vi "Emulator.vi"() -> ()   [LabVIEW 2014]
uses:
  <vilib>/Utility/file.llb/Read From Spreadsheet File (string).vi
panel:
  out "Error Out":errorcluster
  in  "Error In":errorcluster
  in  "Write Loop stop":bool
  in  "file path (dialog if empty)":path=path "C:/Ehsan Temp Folder/TFS/LV/Data Logging with LabVIEW/SV names.csv"
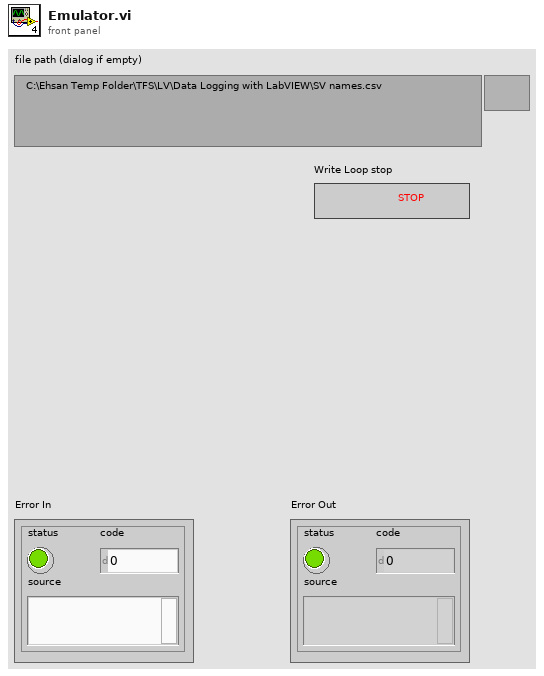
[diagram p1: front panel]
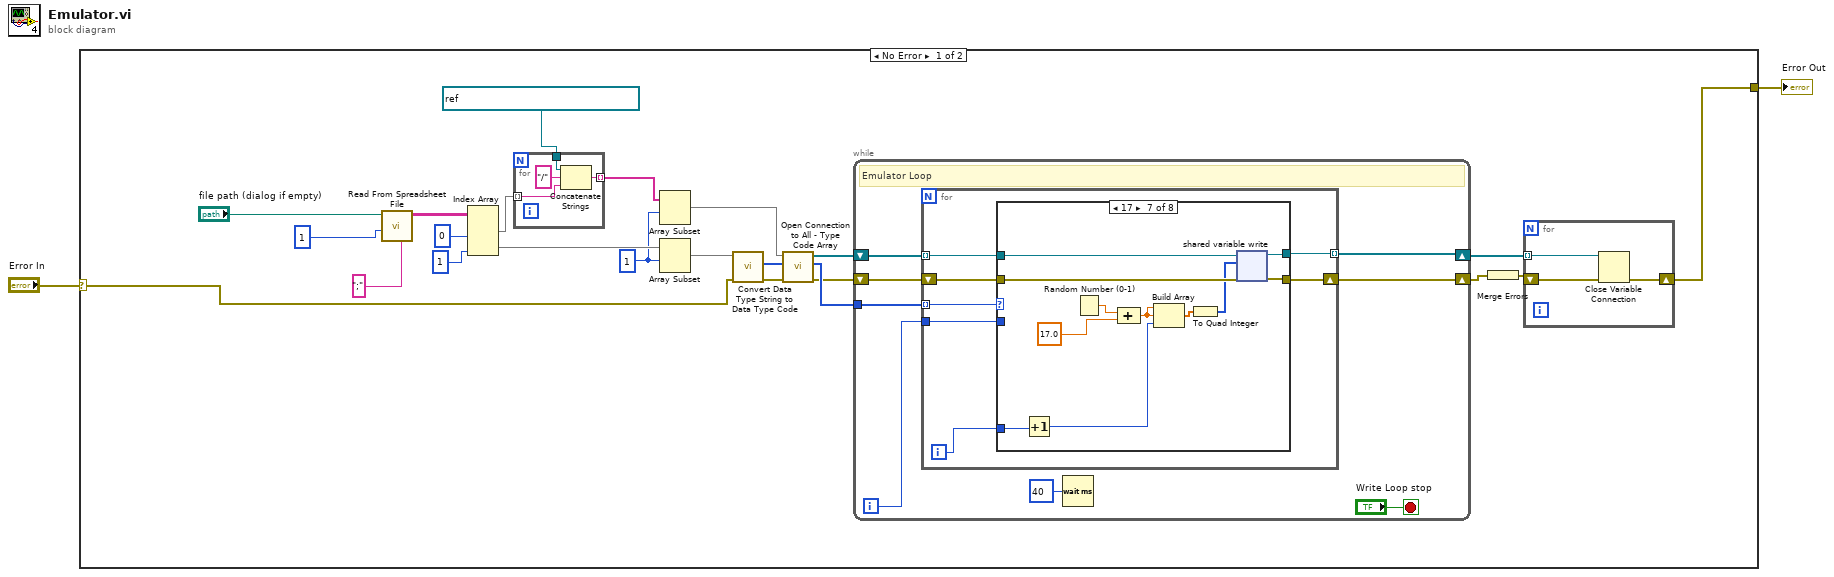
[diagram p0: block diagram]
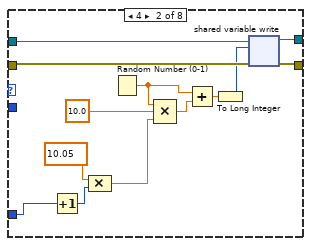
[diagram p3: hidden frame]
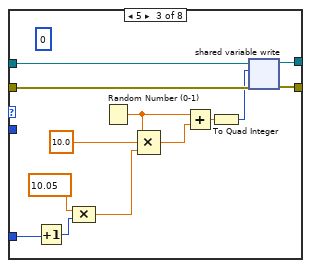
[diagram p4: hidden frame]
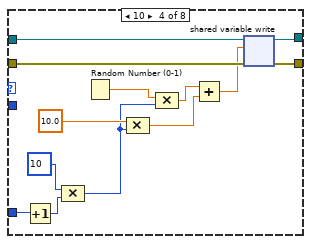
[diagram p5: hidden frame]
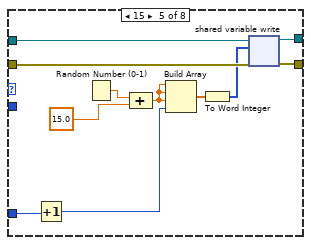
[diagram p6: hidden frame]
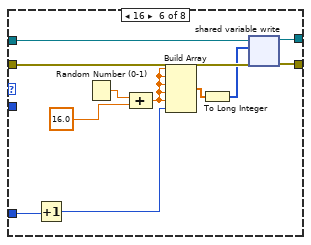
[diagram p7: hidden frame]
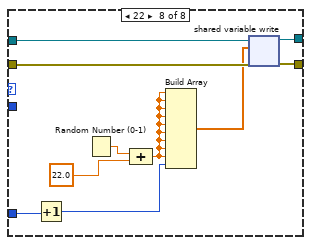
[diagram p8: hidden frame]
diagram:
  n1 = case shown="No Error" "Error In" {
    selector: "Error In" -> [w14 w132]
    tunnel: [w22 w132] -> w1
    frame No Error {
      w5 = 1 ("index")
      n2 = call-poly <vilib>:"Read From Spreadsheet File.vi"("delimiter (\\t)"=";" ("delimiter (\\t)"), "start of read offset (chars.:0)"=1 ("number of rows (all:-1)"), "file path (dialog if empty)"="file path (dialog if empty)") -> ("all rows"=w19:string[][])  [unwired: 4 in, 4 out]
      n3 = Index Array(array=w19, index (col) #1=0 ("index"), index (col) #2=1 ("index")) -> (element #1=w17:string[], element #2=w7:string[])  [unwired: 2 in]
      n4 = for {
        tunnel: w17 -> [w28] mode=indexing
        tunnel: refnum<k21> "ni.var.psp://localhost/test" ("shared variable refnum in") -> [w27]
        tunnel: [w26] -> w4 mode=indexing
        n5 = Concatenate Strings(w27, "/" ("string"), w28) -> (w26:string)
      }
      n6 = Array Subset(array=w4, index=w5) -> (w3:string[])  [unwired: 1 in]
      n7 = Array Subset(array=w7, index=w5) -> (w6:string[])  [unwired: 1 in]
      n8 = call "Convert Data Type String to Data Type Code.vi"("Error In"=w14, "Type Array"=w6) -> ("Error Out"=w13:errorcluster, "Type code Array"=w9:i32[])  [unwired: 7 in, 1 out]
      n9 = call "Open Connection to All - Type Code Array.vi"("Error In"=w13, "Type code Array"=w9, "URL array"=w3) -> ("Error Out"=w10:errorcluster, "Type code Array"=w11:i32[], "Array of SV Refnums"=w12:refnum<k21>[])  [unwired: 5 in, 1 out]
      n10 = while {
        shift-right: [w34] -> w20
        shift-left: w10 -> [w37]
        tunnel: w11 -> [w36]
        shift-right: [w35] -> w23
        shift-left: w12 -> [w38]
        i -> [w33]
        stop <- "Write Loop stop" stop-if-true
        # "Emulator Loop"
        n11 = for {
          tunnel: w38 -> [w47] mode=indexing
          tunnel: w36 -> [w45] mode=indexing
          tunnel: [w44] -> w35 mode=indexing
          shift-right: [w43] -> w34
          shift-left: w37 -> [w46]
          tunnel: w33 -> [w41]
          i -> [w42]
          n12 = case shown="17" w45 {
            tunnel: w47 -> [w49 w62 w75 w88 w99 w110 w121 w131]
            tunnel: w46 -> [w48 w61 w74 w87 w98 w109 w120 w130]
            tunnel: [w49 w59 w72 w86 w96 w107 w118 w128] -> w44
            tunnel: [w48 w60 w73 w85 w97 w108 w119 w129] -> w43
            tunnel: w42 -> [_ w54 w67 w83 w94 w105 w116 w126]
            tunnel: w41 -> [_ _ _ _ _ _ _ _]
            frame -1, Default {
            }
            frame 4 {
              n13 = Increment(x=w54) -> (x+1=w56:i32)
              n14 = Compound Arithmetic op=MULTIPLY(10.05, w56) -> (w55:dbl)
              n15 = Random Number (0-1)() -> (number: 0 to 1=w50:dbl)
              n16 = Compound Arithmetic op=MULTIPLY(w50, 10.0, w55) -> (w53:dbl)
              n17 = Add(x=w50, y=w53) -> (x+y=w52:dbl)
              n18 = To Long Integer(number=w52) -> (32bit integer=w51:i32)
              n19 = shared-variable-write(w62, w61, w51) -> (w59:refnum<k21>, w60:errorcluster)
            }
            frame 5 {
              (unwired) i64 0
              n20 = Increment(x=w67) -> (x+1=w69:i32)
              n21 = Compound Arithmetic op=MULTIPLY(10.05, w69) -> (w68:dbl)
              n22 = Random Number (0-1)() -> (number: 0 to 1=w63:dbl)
              n23 = Compound Arithmetic op=MULTIPLY(w63, 10.0, w68) -> (w66:dbl)
              n24 = Add(x=w63, y=w66) -> (x+y=w65:dbl)
              n25 = To Quad Integer(1:w65) -> (0:w64:i64)
              n26 = shared-variable-write(w75, w74, w64) -> (w72:refnum<k21>, w73:errorcluster)
            }
            frame 10 {
              n27 = Increment(x=w83) -> (x+1=w81:i32)
              n28 = Compound Arithmetic op=MULTIPLY(i64 10, w81) -> (w76:i64)
              n29 = Random Number (0-1)() -> (number: 0 to 1=w78:dbl)
              n30 = Compound Arithmetic op=MULTIPLY(10.0, w76) -> (w80:dbl)
              n31 = Compound Arithmetic op=MULTIPLY(w78, w76) -> (w77:dbl)
              n32 = Add(x=w77, y=w80) -> (x+y=w82:dbl)
              n33 = shared-variable-write(w88, w87, w82) -> (w86:refnum<k21>, w85:errorcluster)
            }
            frame 15 {
              n34 = Increment(x=w94) -> (x+1=w91:i32)
              n35 = Random Number (0-1)() -> (number: 0 to 1=w90:dbl)
              n36 = Compound Arithmetic op=ADD(w90, 15.0) -> (w89:dbl)
              n37 = Build Array(w89, w89, w89, w91) -> (w93:dbl[])
              n38 = To Word Integer(number=w93) -> (16bit integer=w92:i16[])
              n39 = shared-variable-write(w99, w98, w92) -> (w96:refnum<k21>, w97:errorcluster)
            }
            frame 16 {
              n40 = Increment(x=w105) -> (x+1=w102:i32)
              n41 = Random Number (0-1)() -> (number: 0 to 1=w101:dbl)
              n42 = Compound Arithmetic op=ADD(w101, 16.0) -> (w100:dbl)
              n43 = Build Array(w100, w100, w100, w100, w100, w102) -> (w104:dbl[])
              n44 = To Long Integer(number=w104) -> (32bit integer=w103:i32[])
              n45 = shared-variable-write(w110, w109, w103) -> (w107:refnum<k21>, w108:errorcluster)
            }
            frame 17 {
              n46 = Increment(x=w116) -> (x+1=w113:i32)
              n47 = Random Number (0-1)() -> (number: 0 to 1=w112:dbl)
              n48 = Compound Arithmetic op=ADD(w112, 17.0) -> (w111:dbl)
              n49 = Build Array(w111, w111, w113) -> (w115:dbl[])
              n50 = To Quad Integer(1:w115) -> (0:w114:i64[])
              n51 = shared-variable-write(w121, w120, w114) -> (w118:refnum<k21>, w119:errorcluster)
            }
            frame 22 {
              n52 = Increment(x=w126) -> (x+1=w125:i32)
              n53 = Random Number (0-1)() -> (number: 0 to 1=w124:dbl)
              n54 = Compound Arithmetic op=ADD(w124, 22.0) -> (w123:dbl)
              n55 = Build Array(w123, w123, w123, w123, w123, w123, w123, w123, w123, w125) -> (w122:dbl[])
              n56 = shared-variable-write(w131, w130, w122) -> (w128:refnum<k21>, w129:errorcluster)
            }
          }
        }
        n57 = Wait (ms)(milliseconds to wait=u32 40) -> ()  [unwired: 1 out]
      }
      n58 = Merge Errors(w20) -> (w21:errorcluster)
      n59 = for {
        tunnel: w23 -> [w32] mode=indexing
        shift-right: [w30] -> w22
        shift-left: w21 -> [w31]
        n60 = Close Variable Connection(8:w31, 11:w32) -> (0:w30:errorcluster)
      }
    }
    frame Error {
    }
  }
  "Error Out" <- w1
